vi "Scan Routine Aging Martina_NOT FINISHED_v1.0.vi"(2 "Cell Area":dbl, 3 "Pixel Set":bool, 4 "Liv/Div":bool) -> (1 "Efficiency":dbl)   [LabVIEW 2011]
uses:
  Sweep Routine v5.0 Folder/Y/DAQ/Condensed Matter/HJSGroup/LabView/Solar Simulator/Archive/Solar Sim v4.0/Global Variables/MeasurementScanDirection.vi
  Sweep Routine v5.0 Folder/Y/DAQ/Condensed Matter/HJSGroup/LabView/Solar Simulator/Archive/Solar Sim v4.0/Global Variables/MainJVGraph.vi
panel:
  in  "Scan Parameters":T1={"Scan Direction\nDU (T), UD (F)"=FALSE, "Maximum Voltage (V)"=2.0, "Minimum Voltage (V)"=1.0, "Stabilization Time (s)"=10.0, "Range Options"=0} {"Range Options" items=["Auto Range", "Semi-Auto Range", "100 uA", "1 mA", "10 mA", "100 mA", "1A"]}
  in  "Input Queue":T2
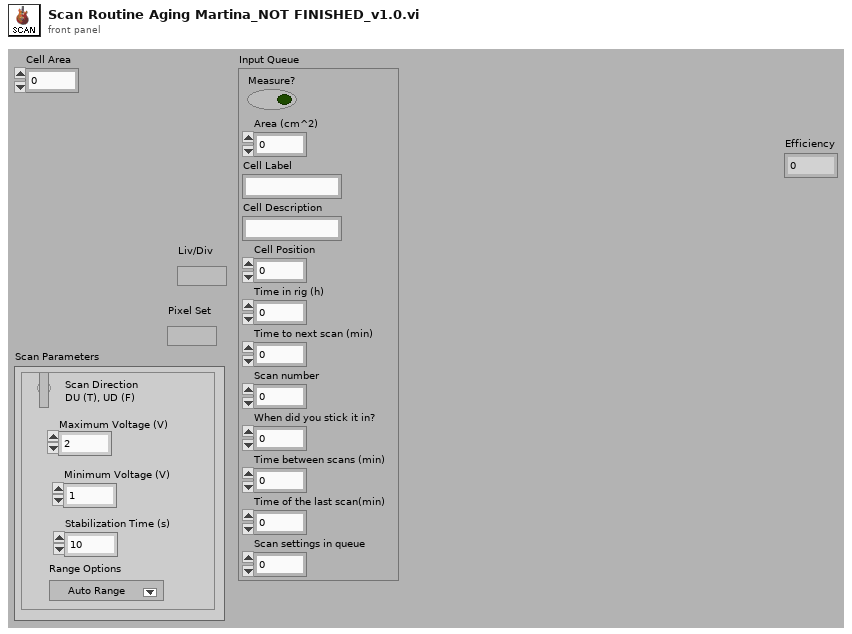
[diagram p1: front panel]
types:
  T1 = cluster{"Scan Direction\nDU (T), UD (F)":bool, "Maximum Voltage (V)":dbl, "Minimum Voltage (V)":dbl, "Stabilization Time (s)":dbl, "Range Options":u16}
  T2 = cluster{"Measure?":bool, "Area (cm^2)":dbl, "Cell Label":string, "Cell Description":string, "Cell Position":i32, "Time in rig (h)":dbl, "Time to next scan (min)":dbl, "Scan number":dbl, "When did you stick it in?":dbl, "Time between scans (min)":dbl, "Time of the last scan(min)":dbl, "Scan settings in queue":u16}
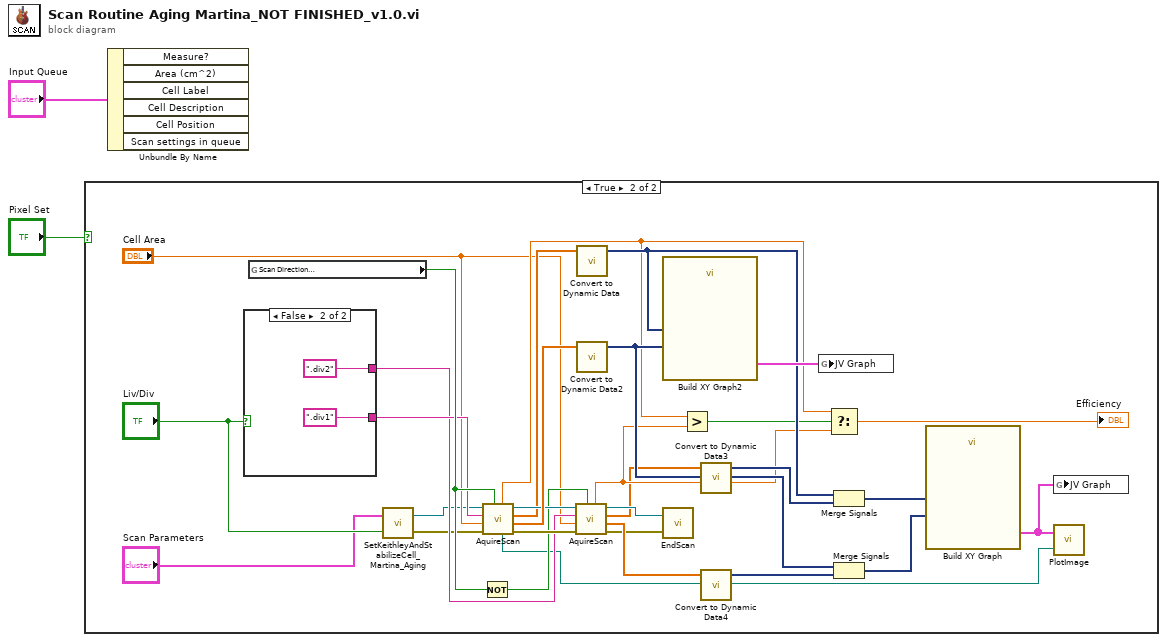
[diagram p0: block diagram]
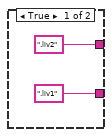
[diagram p3: hidden frame]
diagram:
  n1 = case shown="True" "Pixel Set" {
    frame False {
    }
    frame True {
      n2 = case shown="False" "Liv/Div" {
        tunnel: [".liv1" ".div1"] -> w11
        tunnel: [".liv2" ".div2"] -> w10
        frame True {
        }
        frame False {
        }
      }
      n3 = global read "MeasurementScanDirection.vi" "Scan Direction\nDU (T), UD (F)"() -> (w18:bool)
      n4 = call "SetKeithleyAndStabilizeCell_Martina_Aging.vi"("Liv/Div"="Liv/Div", "Scan Parameters"="Scan Parameters") -> ("error out"=w5:errorcluster, "VISA resource name out"=w6:refnum<visa-resource-name>)
      n5 = Not(x=w18) -> (.not. x?=w17:bool)
      n6 = call "AquireScan.vi"("VISA resource name"=w6, "Extension"=w11, "Cell Area"="Cell Area", "error in (no error)"=w5, "Scan Direction"=w18) -> ("Efficiency"=w15:dbl, "Image Path"=w9:path, "VISA resource name out"=w24:refnum<visa-resource-name>, "V out"=w19:dbl[], "J Out"=w25:dbl[], "error out"=w23:errorcluster)
      n7 = call "AquireScan.vi"("VISA resource name"=w24, "Extension"=w10, "Cell Area"="Cell Area", "error in (no error)"=w23, "Scan Direction"=w17) -> ("Efficiency"=w14:dbl, "VISA resource name out"=w21:refnum<visa-resource-name>, "V out"=w12:dbl[], "J Out"=w22:dbl[], "error out"=w20:errorcluster)  [unwired: 1 out]
      n8 = call "Convert to Dynamic Data"("Array"=w19) -> ("Dynamic Data Type"=w27:dynamicdata)  [unwired: 3 in]
      n9 = call "Convert to Dynamic Data2"("Array"=w25) -> ("Dynamic Data Type"=w26:dynamicdata)  [unwired: 3 in]
      n10 = call "Build XY Graph2"("Y Input"=w26, "X Input"=w27) -> ("XY Graph"=w28:cluster{"Y":dbl[], "Y":dbl[]}[])  [unwired: 8 in, 1 out]
      n11 = call "EndScan.vi"("error in (no error)"=w20, "VISA resource name"=w21) -> ()
      n12 = Greater?(x=w15, y=w14) -> (0:w16:bool)
      n13 = call "Convert to Dynamic Data3"("Array"=w12) -> ("Dynamic Data Type"=w31:dynamicdata)  [unwired: 3 in]
      n14 = call "Convert to Dynamic Data4"("Array"=w22) -> ("Dynamic Data Type"=w29:dynamicdata)  [unwired: 3 in]
      n15 = global write "MainJVGraph.vi" "JV Graph"(w28) -> ()
      n16 = Select(t=w15, s=w16, f=w14) -> (s? t:f=→"Efficiency":dbl)
      n17 = Merge Signals(w27, w31) -> (w32:dynamicdata)
      n18 = Merge Signals(w26, w29) -> (w30:dynamicdata)
      n19 = call "Build XY Graph"("Y Input"=w30, "X Input"=w32) -> ("XY Graph"=w8:cluster{"Y":dbl[], "Y":dbl[]}[])  [unwired: 8 in, 1 out]
      n20 = global write "MainJVGraph.vi" "JV Graph"(w8) -> ()
      n21 = call "PlotImage.vi"("Image Path"=w9, "JV Curves"=w8) -> ()
    }
  }
  n22 = Unbundle By Name("Input Queue") -> ()  [unwired: 6 out]
